vi "Two Buttons.vi"(8 "Button 2 motor speed":dbl, 9 "Button 1":bool, 10 "Button 1 motor speed":dbl, 11 "Button 2":bool) -> (3 "Motor Output":dbl)   [LabVIEW 2015]
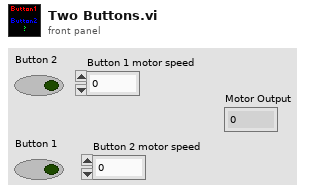
[diagram p1: front panel]
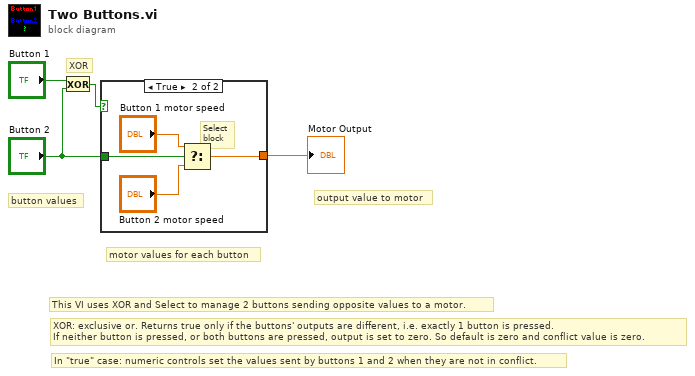
[diagram p0: block diagram]
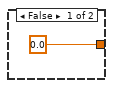
[diagram p2: hidden frame]
diagram:
  # "button values"
  # "output value to motor"
  # "motor values for each button"
  # "In \"true\" case: numeric controls set the values sent by buttons 1 and 2 when they are not in conflict."
  # "XOR"
  # "XOR: exclusive or. Returns true only if the buttons' outputs are different, i.e. exactly 1 button is pressed.\nIf neither button is pressed, or both buttons are pressed, output is set to zero. So default is zero and conflict value is zero."
  # "This VI uses XOR and Select to manage 2 buttons sending opposite values to a motor."
  n1 = Exclusive Or(1:"Button 2", 2:"Button 1") -> (0:w4:bool)
  n2 = case shown="True" w4 {
    tunnel: "Button 2" -> [_ w9]
    tunnel: [0.0 w8] -> w3
    frame False {
    }
    frame True {
      # "Select\nblock"
      n3 = Select(t="Button 1 motor speed", s=w9, f="Button 2 motor speed") -> (s? t:f=w8:dbl)
    }
  }
  "Motor Output" <- w3
